vi "Resonance_FFT.vi"(6 "Start Offset":dbl, 7 "Index":i32, 8 "error in":errorcluster, 9 "dF":dbl, 10 "Length":i32, 11 "Waveform":waveform(dbl)) -> (0 "error out":errorcluster, 1 "Phase":dbl, 2 "Frequency":dbl, 3 "Amplitude":dbl)   [LabVIEW 2023, in "Resonance.lvlib"]
doc: "Computes FFT and then get subset in order to measure the Amplitude, Frequency and Phase of the Resonance in a smaller range"
uses:
  Resonance.lvlib
  <vilib>/Analysis/2dsp.llb/Real FFT.vi
  <vilib>/Analysis/NI_AALPro.lvlib
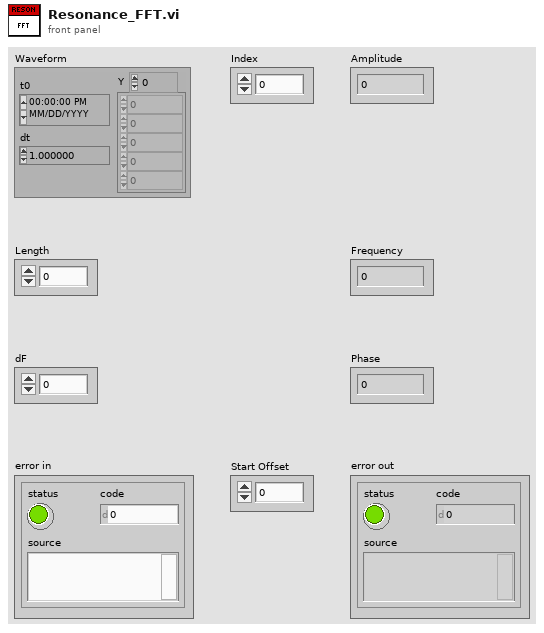
[diagram p1: front panel]
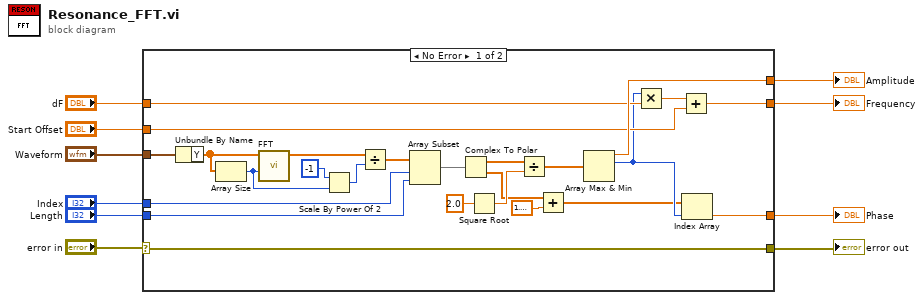
[diagram p0: block diagram]
diagram:
  n1 = case shown="No Error" "error in" {
    selector: "error in" -> [w11 w36]
    tunnel: [w35 _] -> w10
    tunnel: [w34 _] -> w9
    tunnel: [w33 _] -> w8
    tunnel: "Length" -> [w32 _]
    tunnel: "Index" -> [w31 _]
    tunnel: "Start Offset" -> [w28 _]
    tunnel: "dF" -> [w27 _]
    tunnel: "Waveform" -> [w21 _]
    tunnel: [w11 w36] -> w1
    frame No Error {
      n2 = Unbundle By Name(w21) -> ("Y"=w22:dbl[])
      n3 = Array Size(array=w22) -> (size(s)=w23:i32)
      n4 = call-poly <vilib>:"FFT.vi"("FFT size"=w23, "X"=w22) -> ("FFT {X}"=w13:cdb[])  [unwired: 8 in, 1 out]
      n5 = Scale By Power Of 2(n=i16 -1, x=w23) -> (x*2^n=w14:i32)
      n6 = Divide(x=w13, y=w14) -> (x/y=w29:cdb[])
      n7 = Array Subset(array=w29, index=w31, length=w32) -> (w30:cdb[])
      n8 = Complex To Polar(r * e^(i*theta)=w30) -> (r=w19:dbl[], theta=w16:dbl[])
      n9 = Square Root(x=2.0) -> (sqrt(x)=w18:dbl)
      n10 = Divide(x=w19, y=w18) -> (x/y=w20:dbl[])
      n11 = Add(x=w16, y=1.5707963267948966 ("x")) -> (x+y=w25:dbl[])
      n12 = Array Max & Min(array=w20) -> (max value=w35:dbl, max index (indices)=w26:i32)  [unwired: 2 out]
      n13 = Multiply(x=w26, y=w27) -> (x*y=w24:dbl)
      n14 = Add(x=w24, y=w28) -> (x+y=w34:dbl)
      n15 = Index Array(array=w25, index=w26) -> (element=w33:dbl)
    }
    frame Error {
    }
  }
  "Amplitude" <- w10
  "Frequency" <- w9
  "Phase" <- w8
  "error out" <- w1
